vi "random-scale-selector.vi"(10 "Scale Notes":bool[][](array[boolean]), 11 "Scale Names":string[](array[string])) -> (2 "Scale Notes":bool[](array[boolean]), 3 "Scale Name":string)   [LabVIEW 2019]
doc: "This VI selects a random musical scale, and outputs the name and notes of the scale. It needs a list of scales and the notes in each scale."
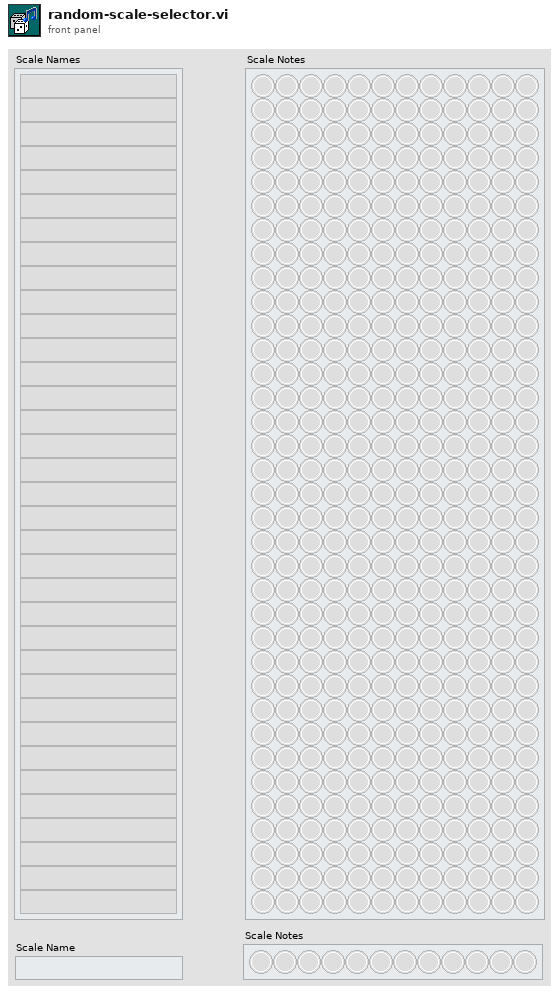
[diagram p1: front panel]
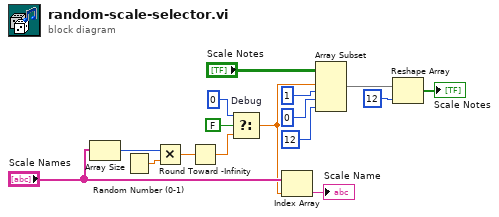
[diagram p0: block diagram]
diagram:
  n1 = Array Size(array="Scale Names") -> (size(s)=w6:i32)
  n2 = Random Number (0-1)() -> (number: 0 to 1=w15:dbl)
  n3 = Multiply(x=w6, y=w15) -> (x*y=w5:dbl)
  n4 = Round Toward -Infinity(1:w5) -> (0:w2:dbl)
  n5 = Select "Debug"(t=0, s=FALSE, f=w2) -> (s? t:f=w1:dbl)
  n6 = Index Array(array="Scale Names", index=w1) -> (element=→"Scale Name":string)
  n7 = Array Subset(array="Scale Notes", index (row)=w1, length (row)=1 ("length"), index (col)=0 ("index"), length (col)=12 ("length")) -> (w12:bool[][])
  n8 = Reshape Array(w12, 12 ("dimension size")) -> (→"Scale Notes":bool[])
